vi "velleman-pl.vi"(0 "Power Control":bool, 3 "isActive":bool) -> (6 "Power Control 2":bool, 7 "Shutter VIS 2":bool, 9 "Shutter UV 2":bool)   [LabVIEW 2015]
uses:
  other/velleman/K8055D.dll
panel:
  out "open":i32
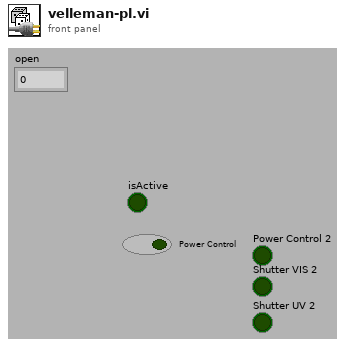
[diagram p1: front panel]
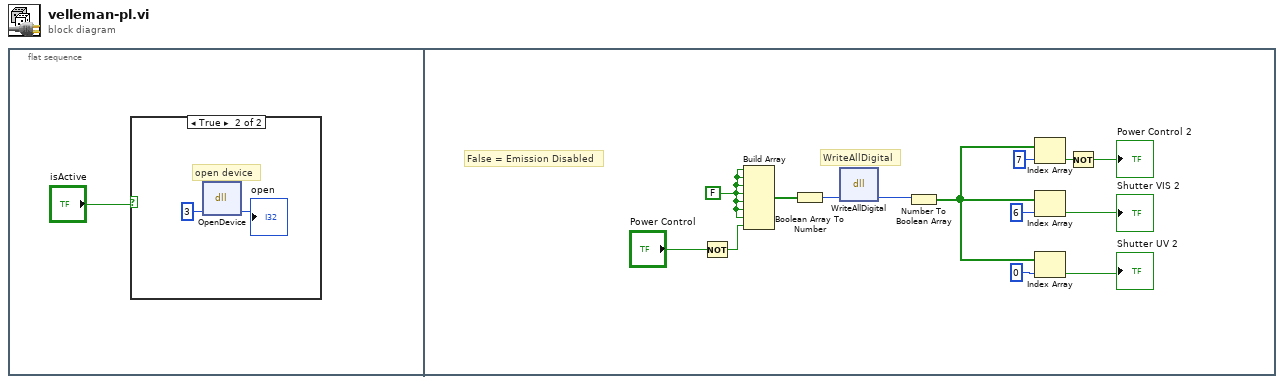
[diagram p0: block diagram]
diagram:
  n1 = flat-sequence {
    frame #0 {
      n2 = case shown="True" "isActive" {
        frame False {
        }
        frame True {
          # "open device"
          n3 = dll-call lib="D:/Programs/LabView/playground/PLEMv3/other/velleman/K8055D.dll" fn="OpenDevice"(3) -> (→"open":i32)  [unwired: 4 in, 2 out]
        }
      }
    }
    frame #1 {
      w5 = FALSE
      # "WriteAllDigital"
      # "False = Emission Disabled"
      n4 = Not(x="Power Control") -> (.not. x?=w4:bool)
      n5 = Build Array(w5, w5, w5, w5, w5, w5, w5, w4) -> (w13:bool[])
      n6 = Boolean Array To Number(Boolean array=w13) -> (number=w12:u32)
      n7 = dll-call lib="D:/Programs/LabView/playground/PLEMv3/other/velleman/K8055D.dll" fn="WriteAllDigital"(w12) -> (w11:i32)  [unwired: 4 in, 2 out]
      n8 = Number To Boolean Array(number=w11) -> (Boolean array=w7:bool[])
      n9 = Index Array(array=w7, index=7) -> (element=w6:bool)
      n10 = Index Array(array=w7, index=6) -> (element=→"Shutter VIS 2":bool)
      n11 = Index Array(array=w7, index=0) -> (element=→"Shutter UV 2":bool)
      n12 = Not(x=w6) -> (.not. x?=→"Power Control 2":bool)
    }
  }
